vi "Event Handler.vi"(0 "uService Template in":refnum<class "Error Manager.lvclass">, 5 "Event type":T1=enum."Message", 7 "Item Name":string, 9 "Data":variant, 11 "error in (no error)":errorcluster) -> (4 "uService Template out":refnum<class "Error Manager.lvclass">, 15 "error out":errorcluster)   [LabVIEW 2026, in "TALOS.lvlib" / "Error Manager.lvlib" / "Error Manager.lvclass"]
doc: "This VI is the event handler of the uService: every time an event is triggered to the uService, this VI is called.\nNote: here you can access the Actor/Class data, but it will be the one coming out from Init. You cannot modify the values.\nThree different events are supported:\nI) Button Pressed: get called on a GUI button pressed. Item Name is the name (label) of the button, Data is empty.\nII) Shared Variable Updated: get called when a SV you subscribed to is updated. Item Name is the name of the SV, and Data is the value (note: you need to convert it to the proper type).\nIII) Message: get called every time a user event is generated using Send Message to Event Handler. The values of Item Name and Data are the one given to the Send Message to Event Handler.\nIV) Ready to launch?: this frame get called every time a new Run is initiated. Each uService is responsible of performing a self check before giving back the green light for the Run to start."
uses:
  Error Manager.lvclass
  C:/LabVIEW Code/TALOS/talos/Father of all uServices/Father of all uServices/Father of all uServices.lvclass
  Father of all uServices/Father of all uServices/Event Handler Items.ctl
  Ancestor/Ancestor/Ancestor.lvclass/Ancestor.ctl
  Error Manager Consumer Case Selector.ctl
  Father of all uServices/Father of all uServices Messages/Consumer Msg/Consumer Msg.lvclass/Consumer Msg.ctl
  Error Info.ctl
  FGV/Error Memory/Get Error Description.vi
  Support VIs/Get PC name.vi
  Ancestor/Ancestor/Read ID.vi
  Support VIs/Get Class Name.vi
  <vilib>/Utility/error.llb/Clear Errors.vi
  Father of all uServices/Father of all uServices Messages/Consumer Msg/Send Consumer.vi
  FGV/Error Memory/Error Memory Core.vi
  <vilib>/AdvancedString/Delimited String to 1D String Array.vi
  <vilib>/AdvancedString/Delimited String to 1D String Array (string).vi
  Support VIs/Circus Root Path.vi
  FGV/Error Memory/Error Crt Lvl checker.vi
  FGV/Error Memory/Error Memory Core.vi/40c8088d-b597-4017-91af-faa98e00292e.vi
  FGV/Error Memory/Error Memory Core.vi/d4a3ab98-063c-4e44-b43d-fbdcfe6c2be2.vi
  Father of all uServices/Father of all uServices/Father of all uServices.lvclass
  C:/LabVIEW Code/TALOS/builds/Actor Framework PPL/Actor Framework.lvlibp/1abvi3w/vi.lib/ActorFramework/Actor/Actor.lvclass
  Support VIs/Global Memory.vi
  <vilib>/Utility/LVClass/Get LV Class Name.vi
  Support VIs/Is in Packed Library.vi
  Support VIs/TALOS Root path.vi
  Support VIs/Read CSV worksheet.vi
  Support VIs/Global Constants.vi
  <vilib>/Utility/error.llb/General Error Handler.vi
  Support VIs/Error Log.vi
  builds/Actor Framework PPL/Actor Framework.lvlibp/1abvi3w/vi.lib/ActorFramework/Actor/Read Self Enqueuer.vi
  <userlib>/_OpenG.lib/lvdata/lvdata.llb/Get Strings from Enum__ogtk.vi
  builds/Actor Framework PPL/Actor Framework.lvlibp/1abvi3w/vi.lib/ActorFramework/Message Enqueuer/Enqueue.vi
  Ancestor/Ancestor/Ancestor.lvclass
  <vilib>/Comparison/Equal/Equal Functor/Equal Functor.lvclass
  Father of all uServices/Father of all uServices Messages/Consumer Msg/Consumer Msg.lvclass
  TALOS.lvlib
  FGV/Error Memory/Error Memory.lvlib
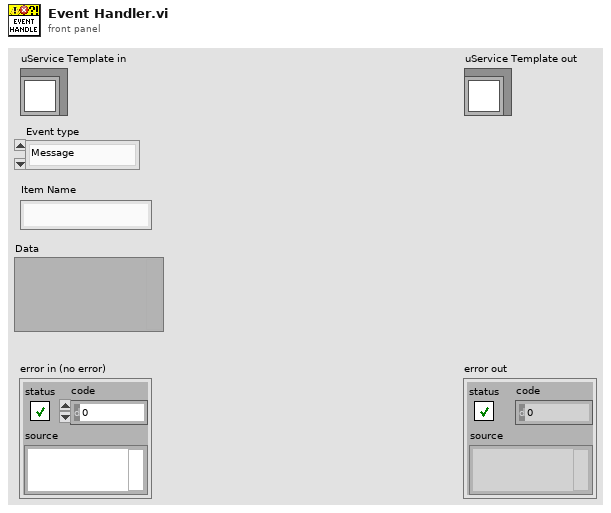
[diagram p1: front panel]
types:
  T1 = typedef "TALOS.lvlib/Father of all uServices.lvlib/Father of all uServices.lvclass/Event Handler Items.ctl" = enum16{"Button Pressed", "Message", "Ready to launch?", "Safe Mode", "Start RUN", "Stop RUN"}
  T2 = typedef "TALOS.lvlib/Error Manager.lvlib/Error Manager.lvclass/Error Manager Consumer Case Selector.ctl" = enum16{"Digest Error", "Dismiss Error", "Dismiss All", "Show Error Details", "Filter out Errors", "Clear Filters", "Check Distributed Mngr Status"}
  T3 = typedef "TALOS.lvlib/Error Manager.lvlib/Error Manager.lvclass/Error Info.ctl" = cluster{"error out":errorcluster, "Time Stamp":timestamp, "Machine Name":string, "GUID":string}
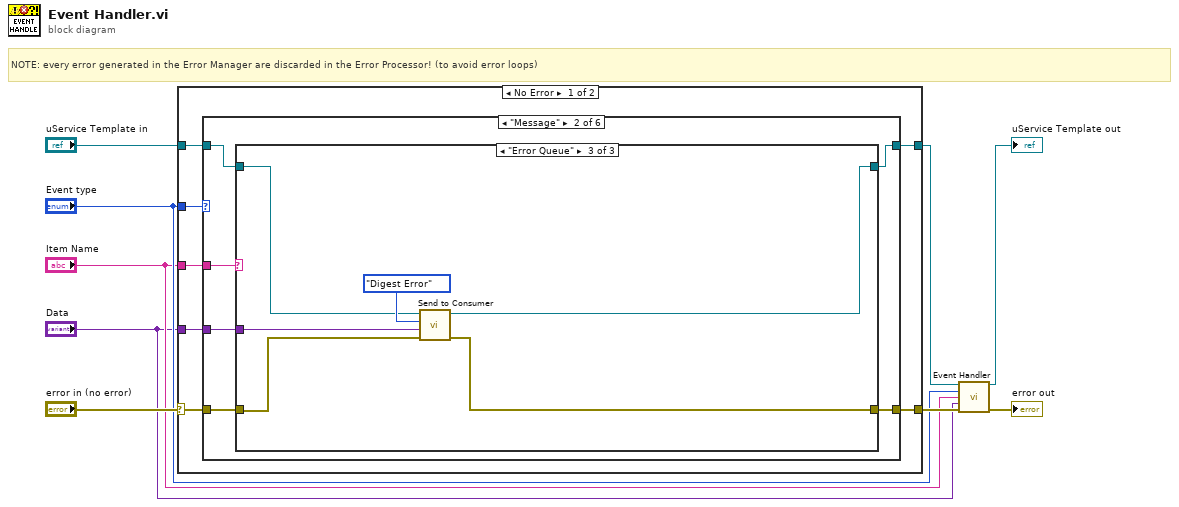
[diagram p0: block diagram]
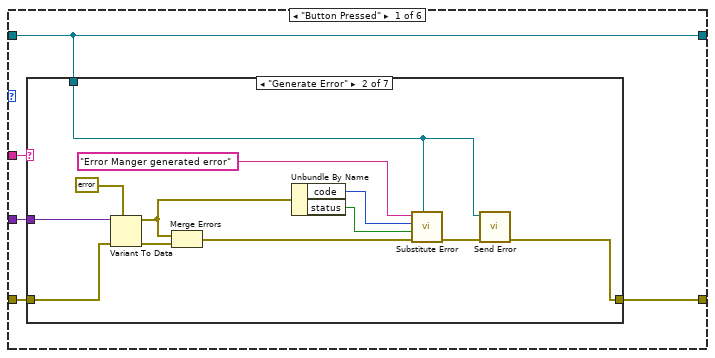
[diagram p2: hidden frame]
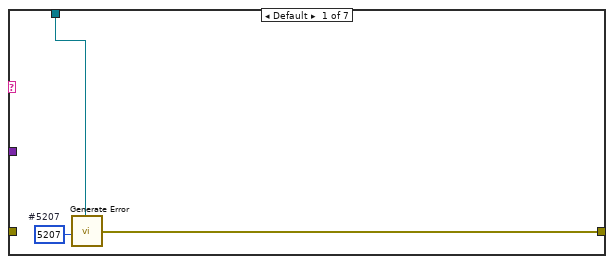
[diagram p3: hidden frame]
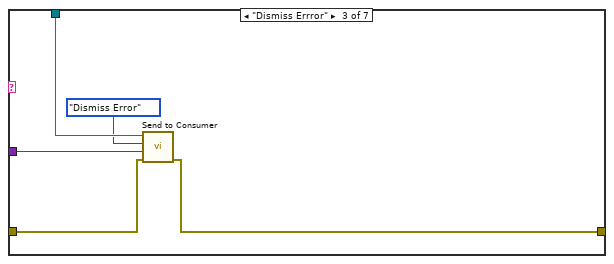
[diagram p4: hidden frame]
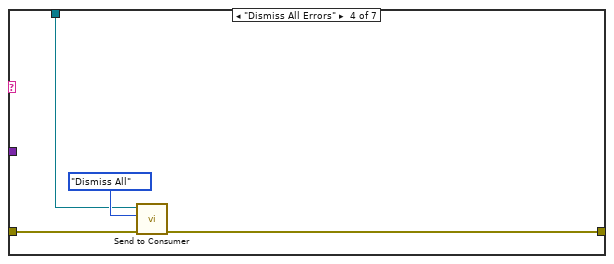
[diagram p5: hidden frame]
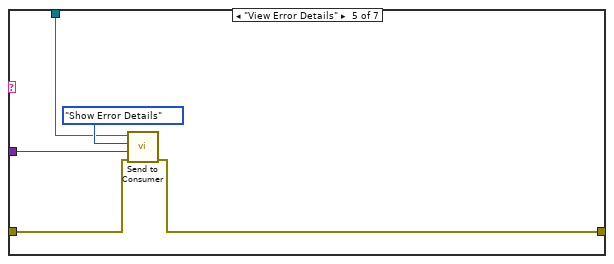
[diagram p6: hidden frame]
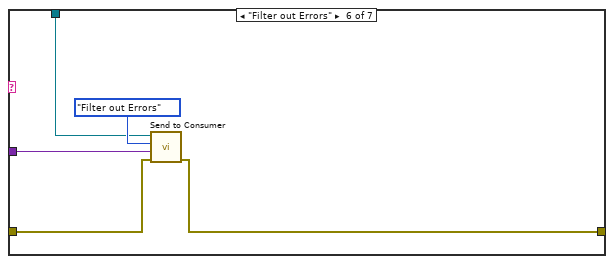
[diagram p7: hidden frame]
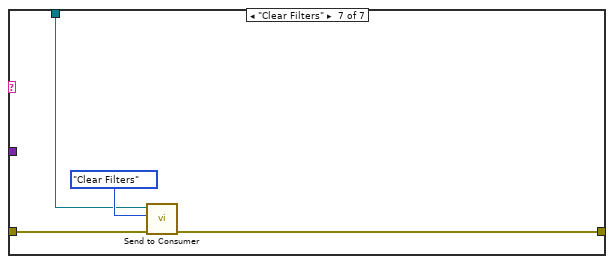
[diagram p8: hidden frame]
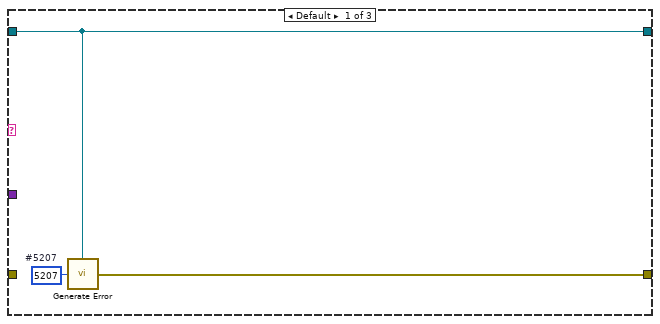
[diagram p9: hidden frame]
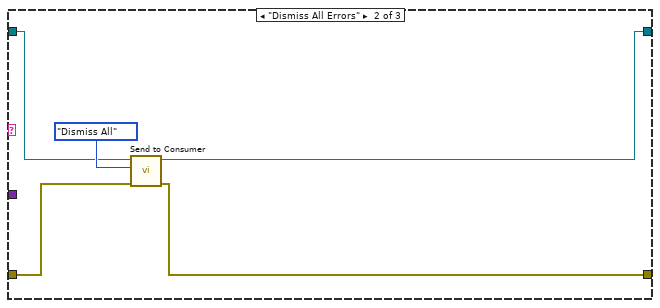
[diagram p10: hidden frame]
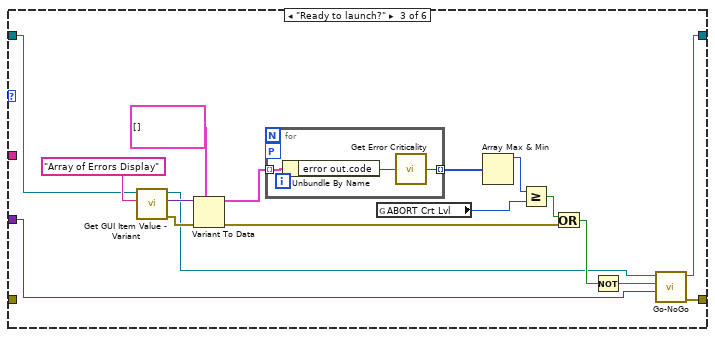
[diagram p11: hidden frame]
diagram:
  # "NOTE: every error generated in the Error Manager are discarded in the Error Processor! (to avoid error loops)"
  n1 = case shown="No Error" "error in (no error)" {
    selector: "error in (no error)" -> [w14 w107]
    tunnel: [w15 w107] -> w7
    tunnel: [w10 w106] -> w4
    tunnel: "uService Template in" -> [w13 w106]
    tunnel: "Event type" -> [w16 _]
    tunnel: "Item Name" -> [w12 _]
    tunnel: "Data" -> [w11 _]
    frame No Error {
      n2 = case shown="\"Message\"" w16 {
        tunnel: [w21 w62 w93 w101 w102 w105] -> w15
        tunnel: w14 -> [w19 w65 _ w101 w102 w105]
        tunnel: w12 -> [w20 w64 _ _ _ _]
        tunnel: w13 -> [w17 w61 w92 w100 w103 w104]
        tunnel: w11 -> [w18 w63 w82 _ _ _]
        tunnel: [w17 w60 w80 w100 w103 w104] -> w10
        frame "Button Pressed" {
          n3 = case shown="\"Generate Error\"" w20 {
            tunnel: w19 -> [_ w34 w39 w43 w48 w53 w57]
            tunnel: [w23 w35 w38 w42 w49 w52 w56] -> w21
            tunnel: w17 -> [w22 w31 w41 w44 w47 w54 w58]
            tunnel: w18 -> [_ w32 w37 _ w46 w51 _]
            frame Default {
              w24 = 5207  # #5207
              n4 = call "Generate Error.vi"("Class"=w22, "Error Code"=w24) -> ("error out"=w23:errorcluster)  [unwired: 5 in]
            }
            frame "Generate Error" {
              n5 = Variant To Data(error in=w34, type=errorcluster {"status"=FALSE, "code"=0, "source"=""} ("error IO"), Variant=w32) -> (data=w28:errorcluster, error out=w36:errorcluster)
              n6 = Merge Errors(w28, w36) -> (w30:errorcluster)
              n7 = Unbundle By Name(w28) -> ("code"=w27:i32, "status"=w26:bool)
              n8 = call "Substitute Error.vi"("LabVIEW Object"=w31, "error in (no error)"=w30, "Error/Warning"=w26, "Error Code"=w27, "Optional String"="Error Manger generated error") -> ("error out"=w29:errorcluster)  [unwired: 6 in]
              n9 = call-dynamic "Send Error.vi"("error in (no error)"=w29, "Father of all uServices in"=w31) -> ("error out"=w35:errorcluster)  [unwired: 8 in, 1 out]
            }
            frame "Dismiss Errror" {
              n10 = call "Send to Consumer.vi"("error in (no error)"=w39, "Data"=w37, "Case ID"=Error_Manager_Consumer_Case_Selector."Dismiss Error" ("ErrMgr Case Selector"), "uService Template in"=w41) -> ("error out"=w38:errorcluster)  [unwired: 6 in, 1 out]
            }
            frame "Dismiss All Errors" {
              n11 = call "Send to Consumer.vi"("error in (no error)"=w43, "Case ID"=Error_Manager_Consumer_Case_Selector."Dismiss All" ("ErrMgr Case Selector"), "uService Template in"=w44) -> ("error out"=w42:errorcluster)  [unwired: 7 in, 1 out]
            }
            frame "View Error Details" {
              n12 = call "Send to Consumer.vi"("error in (no error)"=w48, "Data"=w46, "Case ID"=Error_Manager_Consumer_Case_Selector."Show Error Details" ("ErrMgr Case Selector"), "uService Template in"=w47) -> ("error out"=w49:errorcluster)  [unwired: 6 in, 1 out]
            }
            frame "Filter out Errors" {
              n13 = call "Send to Consumer.vi"("error in (no error)"=w53, "Data"=w51, "Case ID"=Error_Manager_Consumer_Case_Selector."Filter out Errors" ("ErrMgr Case Selector"), "uService Template in"=w54) -> ("error out"=w52:errorcluster)  [unwired: 6 in, 1 out]
            }
            frame "Clear Filters" {
              n14 = call "Send to Consumer.vi"("error in (no error)"=w57, "Case ID"=Error_Manager_Consumer_Case_Selector."Clear Filters" ("ErrMgr Case Selector"), "uService Template in"=w58) -> ("error out"=w56:errorcluster)  [unwired: 7 in, 1 out]
            }
          }
        }
        frame "Message" {
          n15 = case shown="\"Error Queue\"" w64 {
            tunnel: w65 -> [_ w73 w76]
            tunnel: w63 -> [_ _ w77]
            tunnel: w61 -> [w66 w70 w75]
            tunnel: [w68 w72 w79] -> w62
            tunnel: [w66 w69 w74] -> w60
            frame Default {
              w67 = 5207  # #5207
              n16 = call "Generate Error.vi"("Class"=w66, "Error Code"=w67) -> ("error out"=w68:errorcluster)  [unwired: 5 in]
            }
            frame "Dismiss All Errors" {
              n17 = call "Send to Consumer.vi"("error in (no error)"=w73, "Case ID"=Error_Manager_Consumer_Case_Selector."Dismiss All" ("ErrMgr Case Selector"), "uService Template in"=w70) -> ("error out"=w72:errorcluster, "uService Template out"=w69:refnum<class "Error Manager.lvclass">)  [unwired: 7 in]
            }
            frame "Error Queue" {
              n18 = call "Send to Consumer.vi"("error in (no error)"=w76, "Data"=w77, "Case ID"=Error_Manager_Consumer_Case_Selector."Digest Error" ("ErrMgr Case Selector"), "uService Template in"=w75) -> ("error out"=w79:errorcluster, "uService Template out"=w74:refnum<class "Error Manager.lvclass">)  [unwired: 6 in]
            }
          }
        }
        frame "Ready to launch?" {
          n19 = call "Get GUI Item Value - Variant.vi"("FP Item Name"="Array of Errors Display", "uService Template in"=w92) -> ("error out"=w91:errorcluster, "Value"=w95:variant, "uService Template out"=w81:refnum<class "Error Manager.lvclass">)  [unwired: 7 in]
          n20 = Variant To Data(error in=w91, type=T3[] [] ("error constant"), Variant=w95) -> (data=w90:T3[], error out=w86:errorcluster)
          n21 = for {
            tunnel: w90 -> [w99] mode=indexing
            workers-P: _ -> [_]
            tunnel: [w97] -> w89 mode=indexing
            n22 = Unbundle By Name(w99) -> ("error out.code"=w98:i32)
            n23 = call "Get Error Criticality.vi"("Error Code in"=w98) -> ("Error Criticality"=w97:u8)  [unwired: 4 in]
          }
          n24 = global read "Global Constants.vi" "ABORT Crt Lvl"() -> (w83:u8)
          n25 = Array Max & Min(array=w89) -> (max value=w88:u8)  [unwired: 3 out]
          n26 = Greater Or Equal?(x=w88, y=w83) -> (x >= y?=w87:bool)
          n27 = Or(x=w87, y=w86) -> (x .or. y?=w84:bool)
          n28 = Not(x=w84) -> (.not. x?=w85:bool)
          n29 = call-dynamic "Go-NoGo.vi"("Go-NoGo Data"=w82, "Go?"=w85, "Father of all uServices in"=w81) -> ("error out"=w93:errorcluster, "Father of all uServices out"=w80:refnum<class "Error Manager.lvclass">)  [unwired: 7 in]
        }
        frame "Safe Mode" {
        }
        frame "Start RUN" {
        }
        frame "Stop RUN" {
        }
      }
    }
    frame Error {
    }
  }
  n30 = call-parent "Event Handler.vi"("uService Template in"=w4, "Event type"="Event type", "Item Name"="Item Name", "Data"="Data", "error in (no error)"=w7) -> ("uService Template out"=→"uService Template out":refnum<class "Error Manager.lvclass">, "error out"=→"error out":errorcluster)  [unwired: 9 in]
